vi "FlukeCSV2Cluster.vi"(8 "error in (no error)":errorcluster, 11 "FlukePath":path) -> (0 "error out":errorcluster, 3 "AllDataArrays":T1 {"DataAnalysisArray"."TimeStamp" format="%^<%.3X\n%x>T"; "ModelDataArray"."FREQUENCY" format="%#_6f"; "ModelDataArray"."TimeStamp" format="%^<%.3X\n%x>T"; "PMUDataArray"."FREQUENCY" format="%#_6f"; "PMUDataArray"."TimeStamp" format="%^<%.3X\n%x>T"})   [LabVIEW 2014]
uses:
  typedefs/CalcAnalysis.ctl
  typedefs/CalcPhasorError.ctl
  typedefs/PmuRawDataCluster.ctl
  typedefs/PhasorRectangular.ctl
  typedefs/PlotDataArrays.ctl
  <vilib>/Utility/file.llb/Read From Spreadsheet File (string).vi
panel:
  in  "TrueDataCluster":T2 {"FREQUENCY" format="%#_6f"; "TimeStamp" format="%^<%.3X\n%x>T"}
  in  "PmuDataCluster":T2 {"FREQUENCY" format="%#_6f"; "TimeStamp" format="%^<%.3X\n%x>T"}
  in  "CalcAnalysis":T4 {"TimeStamp" format="%^<%.3X\n%x>T"}
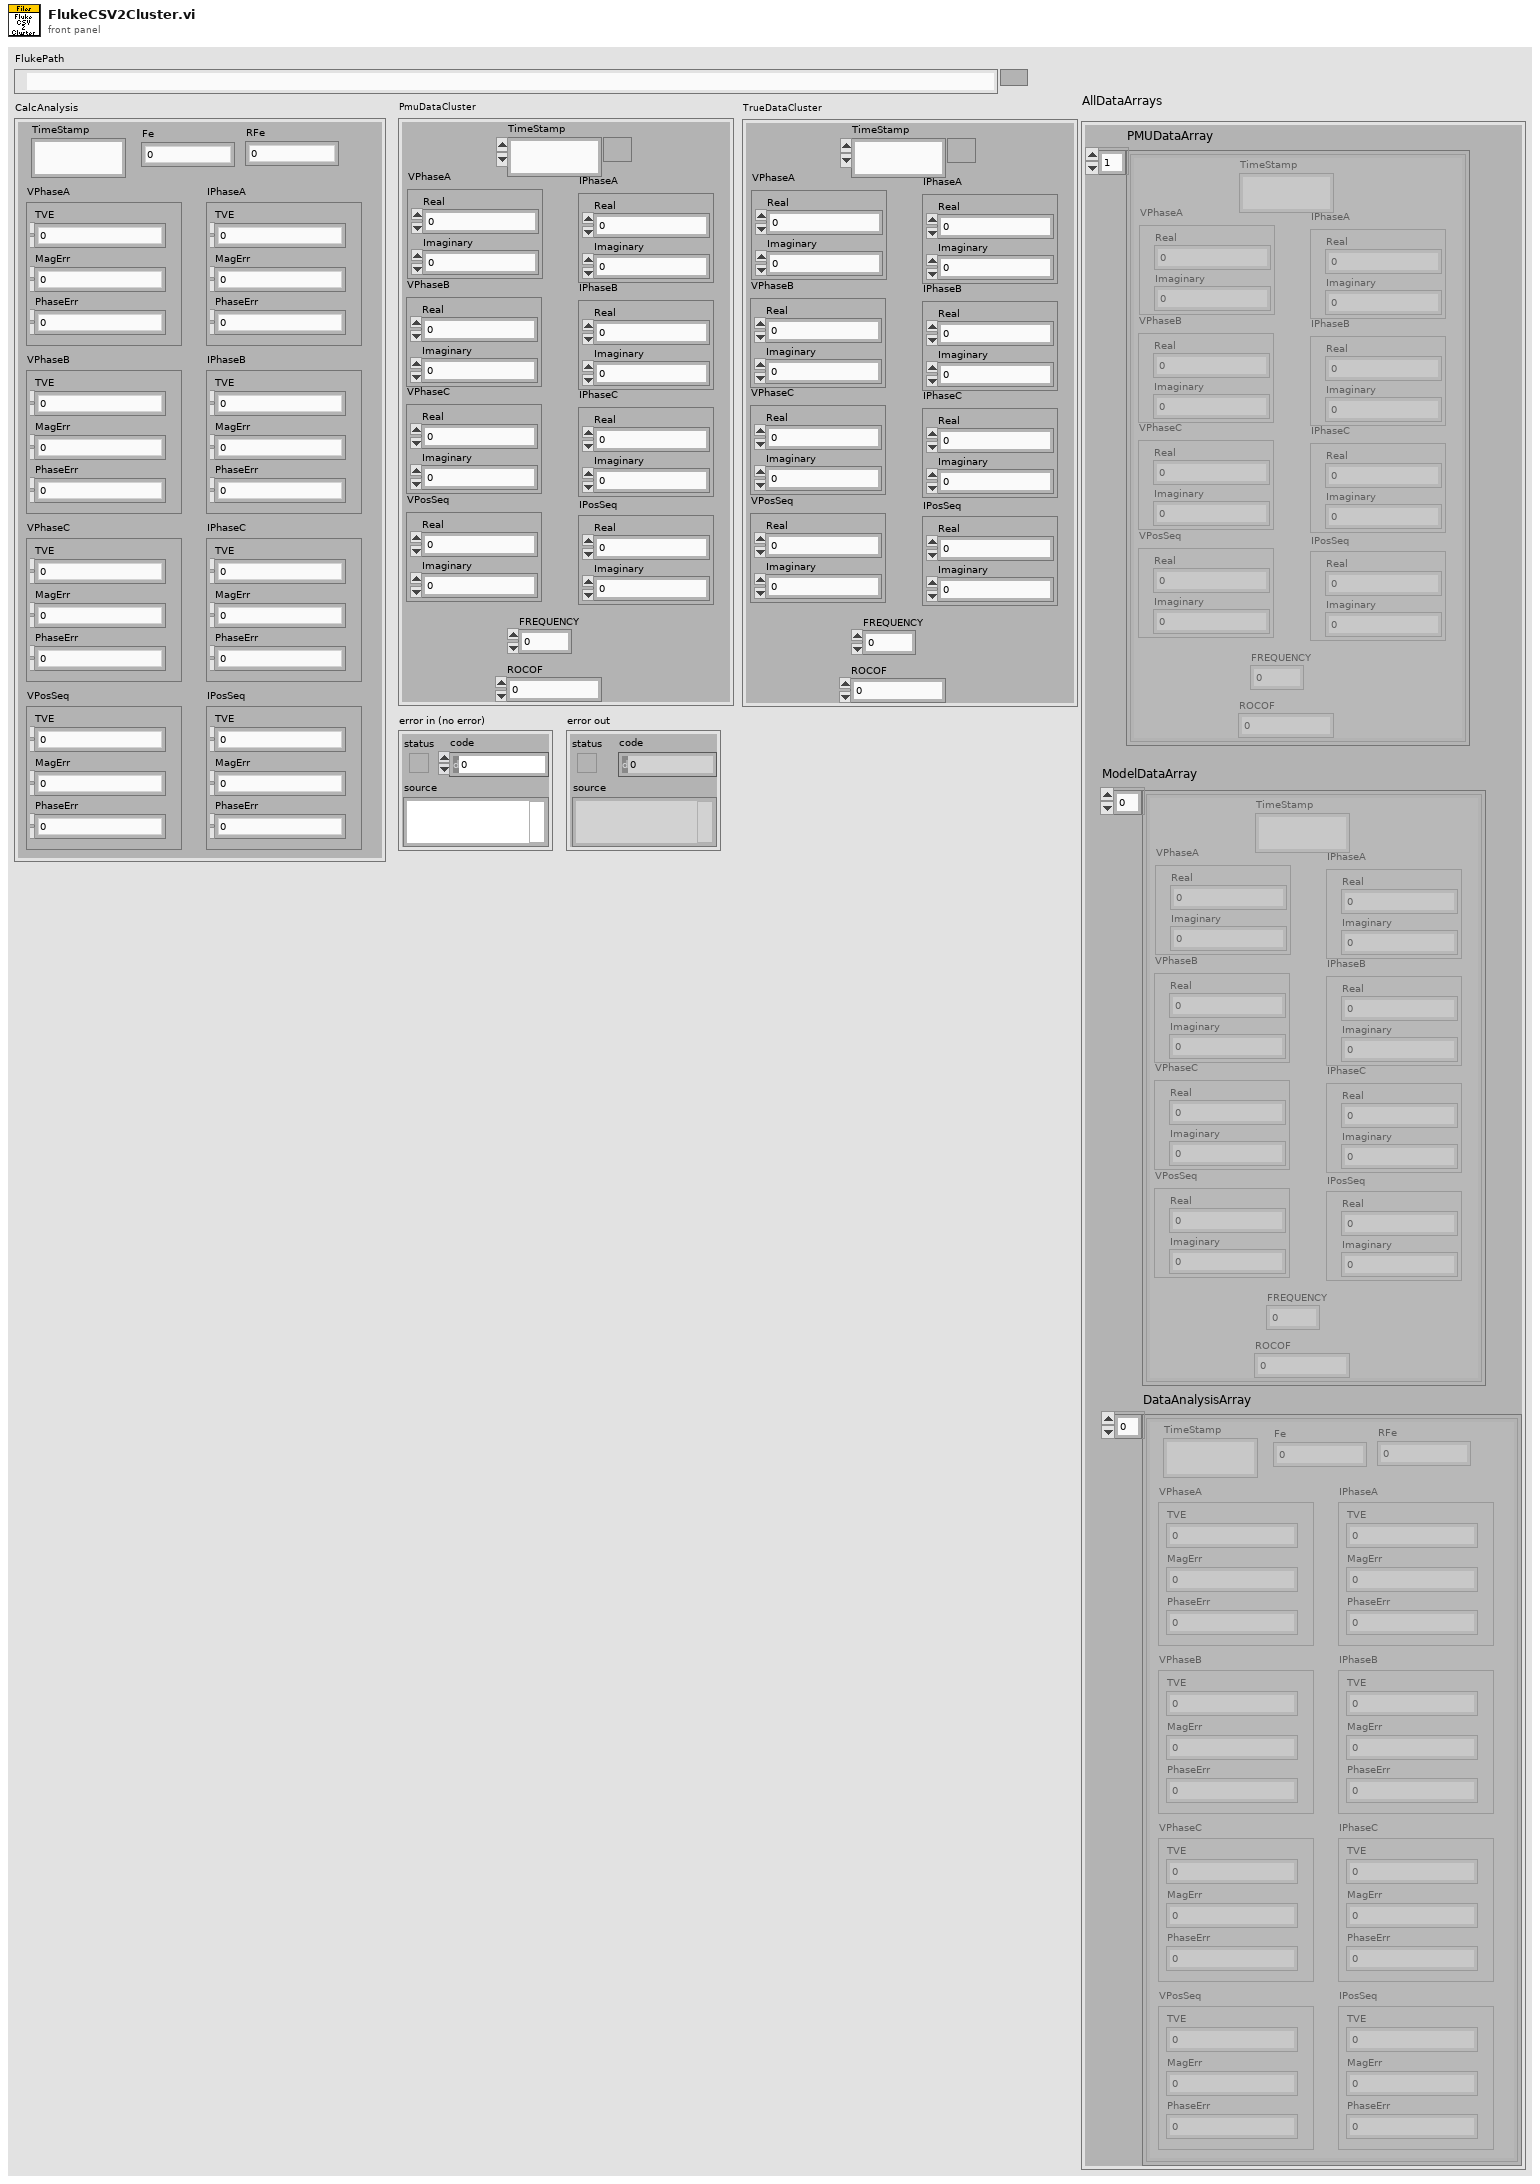
[diagram p1: front panel]
types:
  T1 = typedef "PlotDataArrays.ctl" = cluster{"PMUDataArray":T2[], "ModelDataArray":T2[], "DataAnalysisArray":T4[]}
  T2 = typedef "PmuRawDataCluster.ctl" = cluster{"TimeStamp":timestamp, "VPhaseA":T3, "VPhaseB":T3, "VPhaseC":T3, "VPosSeq":T3, "IPhaseA":T3, "IPhaseB":T3, "IPhaseC":T3, "IPosSeq":T3, "FREQUENCY":dbl, "ROCOF":sgl}
  T3 = typedef "PhasorRectangular.ctl" = cluster{"Real":dbl, "Imaginary":dbl}
  T4 = typedef "CalcAnalysis.ctl" = cluster{"TimeStamp":timestamp, "VPhaseA":T5, "VPhaseB":T5, "VPhaseC":T5, "VPosSeq":T5, "IPhaseA":T5, "IPhaseB":T5, "IPhaseC":T5, "IPosSeq":T5, "Fe":dbl, "RFe":dbl}
  T5 = typedef "CalcPhasorError.ctl" = cluster{"TVE":dbl, "MagErr":dbl, "PhaseErr":dbl}
  T6 = cluster{"TimeStamp":timestamp, "VPhaseA":T3, "VPhaseB":T3, "VPhaseC":T3, "VPosSeq":T3, "IPhaseA":T3, "IPhaseB":T3, "IPhaseC":T3, "IPosSeq":T3, "FREQUENCY":dbl, "ROCOF":sgl}
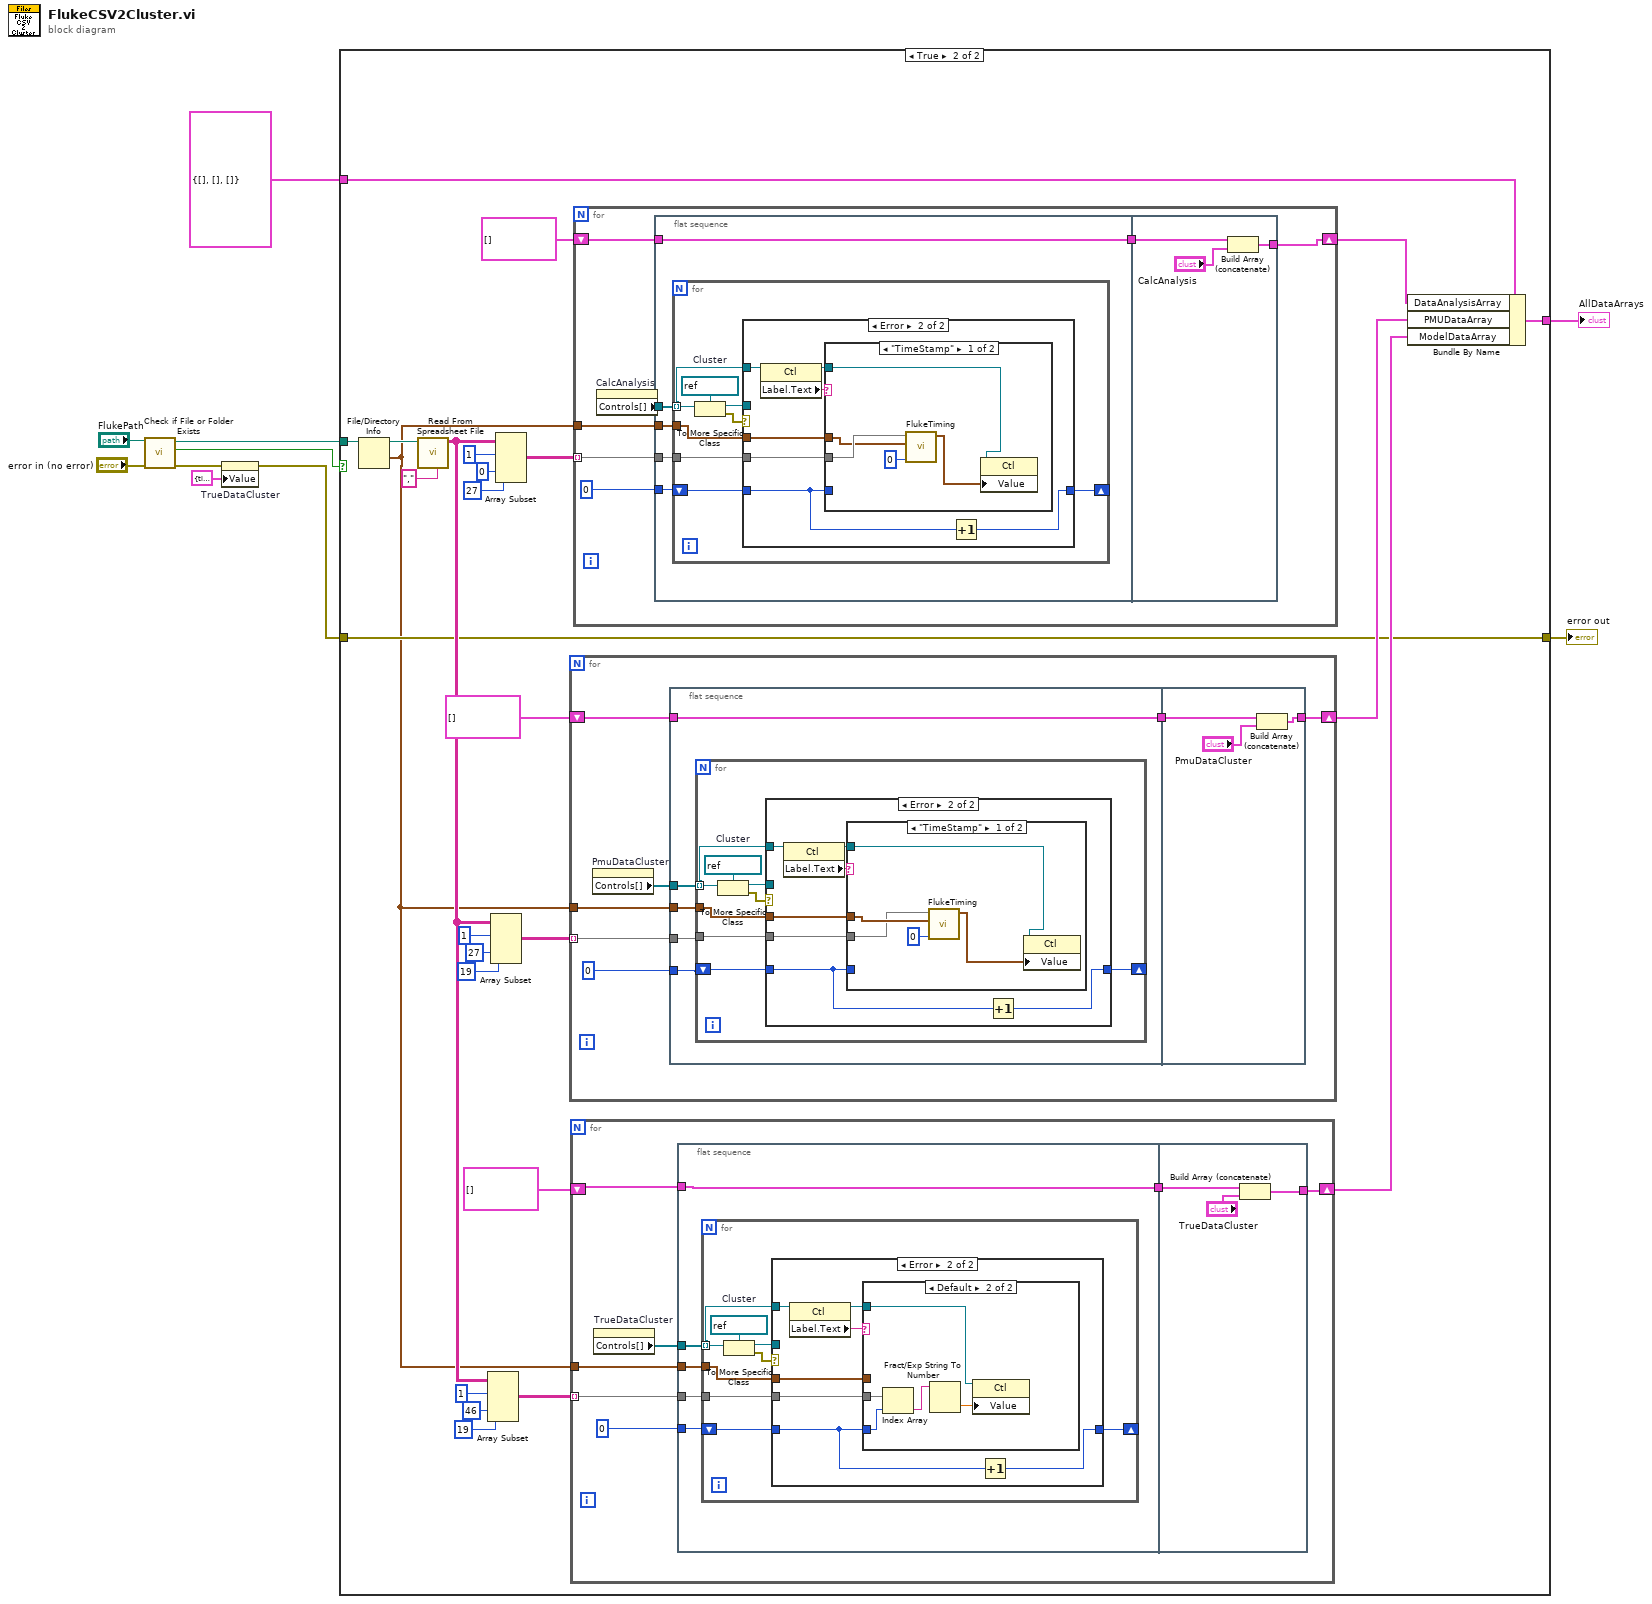
[diagram p0: block diagram]
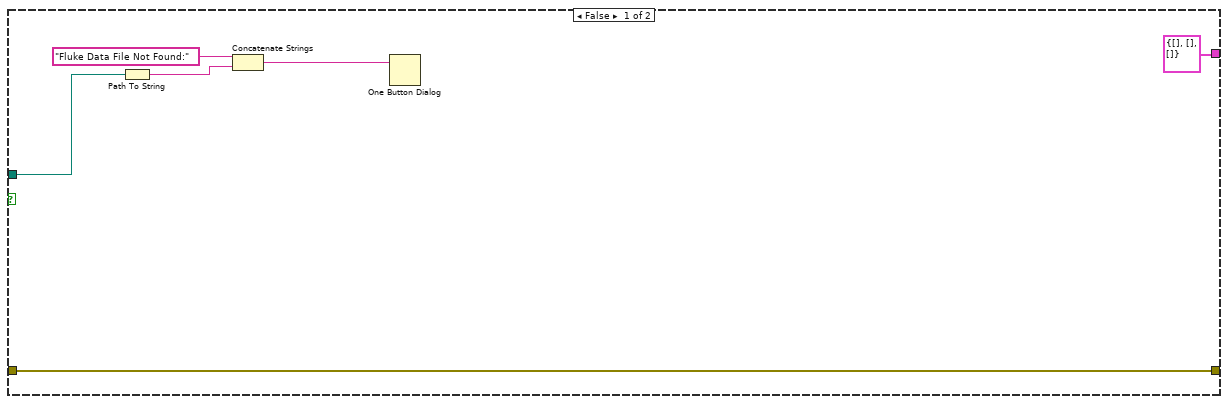
[diagram p2: hidden frame]
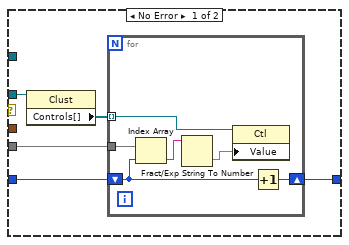
[diagram p3: hidden frame]
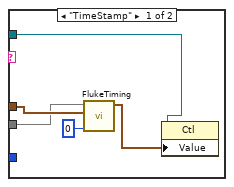
[diagram p4: hidden frame]
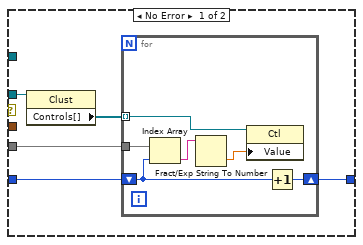
[diagram p5: hidden frame]
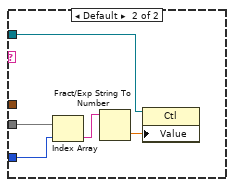
[diagram p6: hidden frame]
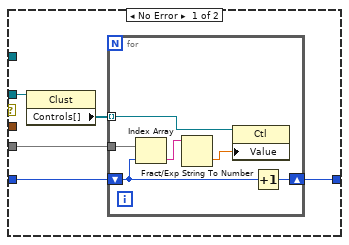
[diagram p7: hidden frame]
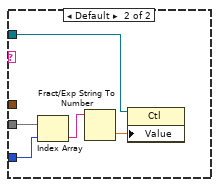
[diagram p8: hidden frame]
diagram:
  n1 = call <vilib>:"Check if File or Folder Exists.vi"("error in (no error)"="error in (no error)", "path"="FlukePath") -> ("error out"=w3:errorcluster, "file or folder exists?"=w7:bool, "dup path"=w8:path)  [unwired: 7 in]
  n2 = property on="TrueDataCluster" class="Clust (strict)"(error in=w3, "Value"=T6 {"TimeStamp"=timestamp(51239 s since 1904-01-01), "VPhaseA"={"Real"=0.0, "Imaginary"=0.0}, "VPhaseB"={"Real"=0.0, "Imaginary"=0.0}, "VPhaseC"={"Real"=0.0, "Imaginary"=0.0}, "VPosSeq"={"Real"=0.0, "Imaginary"=0.0}, "IPhaseA"={"Real"=0.0, "Imaginary"=0.0}, "IPhaseB"={"Real"=0.0, "Imaginary"=0.0}, "IPhaseC"={"Real"=0.0, "Imaginary"=0.0}, "IPosSeq"={"Real"=0.0, "Imaginary"=0.0}, "FREQUENCY"=0.0, "ROCOF"=0.0}) -> (error out=w2:errorcluster)  [unwired: 1 in, 1 out]
  n3 = case shown="True" w7 {
    tunnel: w8 -> [w14 w23]
    tunnel: w2 -> [w11 w24]
    tunnel: [T1 {"PMUDataArray"=[], "ModelDataArray"=[], "DataAnalysisArray"=[]} ("AllDataArrays") w25] -> w6
    tunnel: [w11 w24] -> w5
    tunnel: T1 {"PMUDataArray"=[], "ModelDataArray"=[], "DataAnalysisArray"=[]} ("AllDataArrays") -> [_ w20]
    frame False {
      n4 = Path To String(path=w14) -> (string=w15:string)
      n5 = Concatenate Strings("Fluke Data File Not Found:", w15) -> (w13:string)
      n6 = One Button Dialog(message=w13) -> ()  [unwired: 1 in, 1 out]
    }
    frame True {
      n7 = File/Directory Info(path=w23) -> (path out=w22:path, last mod=w21:timestamp)  [unwired: 1 in, 5 out]
      n8 = call-poly <vilib>:"Read From Spreadsheet File.vi"("delimiter (\\t)"="," ("delimiter (\\t)"), "file path (dialog if empty)"=w22) -> ("all rows"=w29:string[][])  [unwired: 5 in, 4 out]
      n9 = Array Subset(array=w29, index (row)=1 ("index"), index (col)=46 ("index"), length (col)=19 ("length")) -> (w30:string[][])  [unwired: 1 in]
      n10 = Array Subset(array=w29, index (row)=1 ("index"), index (col)=27 ("index"), length (col)=19 ("length")) -> (w37:string[][])  [unwired: 1 in]
      n11 = Array Subset(array=w29, index (row)=1 ("index"), index (col)=0 ("index"), length (col)=27 ("length")) -> (w38:string[][])  [unwired: 1 in]
      n12 = for {
        tunnel: w37 -> [w99] mode=indexing
        tunnel: w21 -> [w97]
        shift-right: [w96] -> w27
        shift-left: T2[] [] -> [w95]
        n13 = property on="PmuDataCluster" class="Clust (strict)"() -> ("Controls[]"=w100:refnum<vi>[])  [unwired: 2 in, 2 out]
        n14 = flat-sequence {
          tunnel: w100 -> [w105]
          tunnel: w99 -> [w104]
          tunnel: 0 ("index") -> [w103]
          tunnel: w97 -> [w102]
          tunnel: w95 -> [w101]
          tunnel: [w101] -> w94
          tunnel: [w143] -> w96
          tunnel: w94 -> [w142]
          frame #0 {
            n15 = for {
              tunnel: w105 -> [w107] mode=indexing
              tunnel: w104 -> [w110]
              shift-right: [w108] -> _
              shift-left: w103 -> [w109]
              tunnel: w102 -> [w106]
              w113 = refnum<vi> refnum  # Cluster
              n16 = To More Specific Class(target class=w113, reference=w107) -> (specific class reference=w111:refnum<vi>, error out=w112:errorcluster)  [unwired: 1 in]
              n17 = case shown="Error" w112 {
                tunnel: w111 -> [w118 _]
                tunnel: w110 -> [w116 w128]
                tunnel: w109 -> [w115 w127]
                tunnel: [w114 w126] -> w108
                tunnel: w107 -> [_ w131]
                tunnel: w106 -> [_ w125]
                frame No Error {
                  n18 = property class="Clust"(reference=w118) -> ("Controls[]"=w117:refnum<vi>[])  [unwired: 1 in, 2 out]
                  n19 = for {
                    tunnel: w117 -> [w121] mode=indexing
                    tunnel: w116 -> [w124]
                    shift-right: [w119] -> w114
                    shift-left: w115 -> [w123]
                    n20 = Index Array(array=w124, index=w123) -> (element=w122:string)
                    n21 = Fract/Exp String To Number(string=w122) -> (number=w120:dbl)  [unwired: 3 in, 1 out]
                    n22 = property class="Ctl"(reference=w121, "Value"=w120) -> ()  [unwired: 1 in, 2 out]
                    n23 = Increment(x=w123) -> (x+1=w119:i32)
                  }
                }
                frame Error {
                  n24 = property class="Ctl"(reference=w131) -> (reference out=w129:refnum<vi>, "Label.Text"=w130:string)  [unwired: 1 in, 1 out]
                  n25 = case shown="\"TimeStamp\"" w130 {
                    tunnel: w129 -> [w136 w138]
                    tunnel: w128 -> [w134 w140]
                    tunnel: w127 -> [_ w141]
                    tunnel: w125 -> [w135 _]
                    frame "TimeStamp" {
                      n26 = call "FlukeTiming.vi"("UTC"=i16 0, "file timestamp"=w135, "array"=w134) -> ("timestamp out"=w132:timestamp)  [unwired: 8 in]
                      n27 = property class="Ctl"(reference=w136, "Value"=w132) -> ()  [unwired: 1 in, 2 out]
                    }
                    frame Default {
                      n28 = Index Array(array=w140, index=w141) -> (element=w139:string)
                      n29 = Fract/Exp String To Number(string=w139) -> (number=w137:dbl)  [unwired: 3 in, 1 out]
                      n30 = property class="Ctl"(reference=w138, "Value"=w137) -> ()  [unwired: 1 in, 2 out]
                    }
                  }
                  n31 = Increment(x=w127) -> (x+1=w126:i32)
                }
              }
            }
          }
          frame #1 {
            n32 = Build Array (concatenate)(w142, "PmuDataCluster") -> (w143:T2[])
          }
        }
      }
      n33 = for {
        tunnel: w30 -> [w48] mode=indexing
        tunnel: w21 -> [w46]
        shift-right: [w45] -> w26
        shift-left: T2[] [] -> [w44]
        n34 = property on="TrueDataCluster" class="Clust (strict)"() -> ("Controls[]"=w49:refnum<vi>[])  [unwired: 2 in, 2 out]
        n35 = flat-sequence {
          tunnel: w49 -> [w54]
          tunnel: w48 -> [w53]
          tunnel: 0 ("index") -> [w52]
          tunnel: w46 -> [w51]
          tunnel: w44 -> [w50]
          tunnel: [w50] -> w43
          tunnel: [w92] -> w45
          tunnel: w43 -> [w91]
          frame #0 {
            n36 = for {
              tunnel: w54 -> [w56] mode=indexing
              tunnel: w53 -> [w59]
              shift-right: [w57] -> _
              shift-left: w52 -> [w58]
              tunnel: w51 -> [w55]
              w62 = refnum<vi> refnum  # Cluster
              n37 = To More Specific Class(target class=w62, reference=w56) -> (specific class reference=w60:refnum<vi>, error out=w61:errorcluster)  [unwired: 1 in]
              n38 = case shown="Error" w61 {
                tunnel: w60 -> [w67 _]
                tunnel: w59 -> [w65 w77]
                tunnel: w58 -> [w64 w76]
                tunnel: [w63 w75] -> w57
                tunnel: w56 -> [_ w80]
                tunnel: w55 -> [_ w74]
                frame No Error {
                  n39 = property class="Clust"(reference=w67) -> ("Controls[]"=w66:refnum<vi>[])  [unwired: 1 in, 2 out]
                  n40 = for {
                    tunnel: w66 -> [w70] mode=indexing
                    tunnel: w65 -> [w73]
                    shift-right: [w68] -> w63
                    shift-left: w64 -> [w72]
                    n41 = Index Array(array=w73, index=w72) -> (element=w71:string)
                    n42 = Fract/Exp String To Number(string=w71) -> (number=w69:dbl)  [unwired: 3 in, 1 out]
                    n43 = property class="Ctl"(reference=w70, "Value"=w69) -> ()  [unwired: 1 in, 2 out]
                    n44 = Increment(x=w72) -> (x+1=w68:i32)
                  }
                }
                frame Error {
                  n45 = property class="Ctl"(reference=w80) -> (reference out=w78:refnum<vi>, "Label.Text"=w79:string)  [unwired: 1 in, 1 out]
                  n46 = case shown="Default" w79 {
                    tunnel: w78 -> [w85 w87]
                    tunnel: w77 -> [w83 w89]
                    tunnel: w76 -> [_ w90]
                    tunnel: w74 -> [w84 _]
                    frame "TimeStamp" {
                      n47 = call "FlukeTiming.vi"("UTC"=i16 0, "file timestamp"=w84, "array"=w83) -> ("timestamp out"=w81:timestamp)  [unwired: 8 in]
                      n48 = property class="Ctl"(reference=w85, "Value"=w81) -> ()  [unwired: 1 in, 2 out]
                    }
                    frame Default {
                      n49 = Index Array(array=w89, index=w90) -> (element=w88:string)
                      n50 = Fract/Exp String To Number(string=w88) -> (number=w86:dbl)  [unwired: 3 in, 1 out]
                      n51 = property class="Ctl"(reference=w87, "Value"=w86) -> ()  [unwired: 1 in, 2 out]
                    }
                  }
                  n52 = Increment(x=w76) -> (x+1=w75:i32)
                }
              }
            }
          }
          frame #1 {
            n53 = Build Array (concatenate)(w91, "TrueDataCluster") -> (w92:T2[])
          }
        }
      }
      n54 = for {
        tunnel: w38 -> [w151] mode=indexing
        tunnel: w21 -> [w149]
        shift-right: [w146] -> w28
        shift-left: T4[] [] -> [w148]
        n55 = property on="CalcAnalysis" class="Clust (strict)"() -> ("Controls[]"=w147:refnum<vi>[])  [unwired: 2 in, 2 out]
        n56 = flat-sequence {
          tunnel: w151 -> [w156]
          tunnel: 0 ("index") -> [w155]
          tunnel: w149 -> [w154]
          tunnel: w148 -> [w152]
          tunnel: w147 -> [w153]
          tunnel: [w152] -> w145
          tunnel: [w195] -> w146
          tunnel: w145 -> [w193]
          frame #0 {
            n57 = for {
              tunnel: w153 -> [w158] mode=indexing
              tunnel: w156 -> [w161]
              shift-right: [w159] -> _
              shift-left: w155 -> [w160]
              tunnel: w154 -> [w157]
              w164 = refnum<vi> refnum  # Cluster
              n58 = To More Specific Class(target class=w164, reference=w158) -> (specific class reference=w162:refnum<vi>, error out=w163:errorcluster)  [unwired: 1 in]
              n59 = case shown="Error" w163 {
                tunnel: w162 -> [w169 _]
                tunnel: w161 -> [w167 w179]
                tunnel: w160 -> [w166 w178]
                tunnel: [w165 w177] -> w159
                tunnel: w158 -> [_ w182]
                tunnel: w157 -> [_ w176]
                frame No Error {
                  n60 = property class="Clust"(reference=w169) -> ("Controls[]"=w168:refnum<vi>[])  [unwired: 1 in, 2 out]
                  n61 = for {
                    tunnel: w168 -> [w172] mode=indexing
                    tunnel: w167 -> [w175]
                    shift-right: [w170] -> w165
                    shift-left: w166 -> [w174]
                    n62 = Index Array(array=w175, index=w174) -> (element=w173:string)
                    n63 = Fract/Exp String To Number(string=w173) -> (number=w171:dbl)  [unwired: 3 in, 1 out]
                    n64 = property class="Ctl"(reference=w172, "Value"=w171) -> ()  [unwired: 1 in, 2 out]
                    n65 = Increment(x=w174) -> (x+1=w170:i32)
                  }
                }
                frame Error {
                  n66 = property class="Ctl"(reference=w182) -> (reference out=w180:refnum<vi>, "Label.Text"=w181:string)  [unwired: 1 in, 1 out]
                  n67 = case shown="\"TimeStamp\"" w181 {
                    tunnel: w180 -> [w187 w189]
                    tunnel: w179 -> [w186 w191]
                    tunnel: w178 -> [_ w192]
                    tunnel: w176 -> [w185 _]
                    frame "TimeStamp" {
                      n68 = call "FlukeTiming.vi"("UTC"=i16 0, "file timestamp"=w185, "array"=w186) -> ("timestamp out"=w183:timestamp)  [unwired: 8 in]
                      n69 = property class="Ctl"(reference=w187, "Value"=w183) -> ()  [unwired: 1 in, 2 out]
                    }
                    frame Default {
                      n70 = Index Array(array=w191, index=w192) -> (element=w190:string)
                      n71 = Fract/Exp String To Number(string=w190) -> (number=w188:dbl)  [unwired: 3 in, 1 out]
                      n72 = property class="Ctl"(reference=w189, "Value"=w188) -> ()  [unwired: 1 in, 2 out]
                    }
                  }
                  n73 = Increment(x=w178) -> (x+1=w177:i32)
                }
              }
            }
          }
          frame #1 {
            n74 = Build Array (concatenate)(w193, "CalcAnalysis") -> (w195:T4[])
          }
        }
      }
      n75 = Bundle By Name(cluster=w20, "DataAnalysisArray"=w28, "PMUDataArray"=w27, "ModelDataArray"=w26) -> (w25:T1)
    }
  }
  "AllDataArrays" <- w6
  "error out" <- w5
